vi "test_MonoAllTests.vi"(7 "Test should pass":bool=TRUE, 8 "error in":errorcluster, 9 "tear down connection":bool=TRUE, 10 "set-up a connection":bool=TRUE, 11 "device selection":enum16{"monochromator", "CCD", "SCD"}(ring)) -> (0 "error out":errorcluster)   [LabVIEW 2023]
uses:
  Classes/CCD/CCD.lvclass
  C:/Projects/Horiba/horiba-labview-sdk/Source/Classes/GenericDevice/GenericDevice.lvclass
  <vilib>/addons/_JKI Toolkits/Caraya/classes/Test/Test.lvclass
  <vilib>/Hampel Software Engineering/HSE Logger/hse-logger.lvlib
panel:
  in  "init mono?":bool
  out "log-file path":path
  # "Connector Pane"
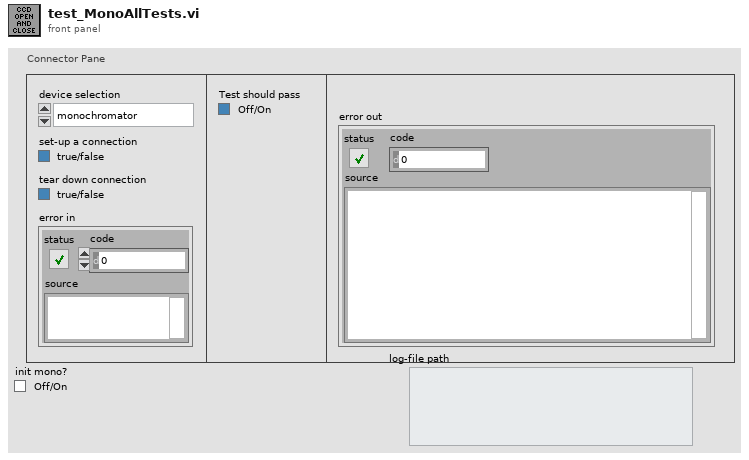
[diagram p1: front panel]
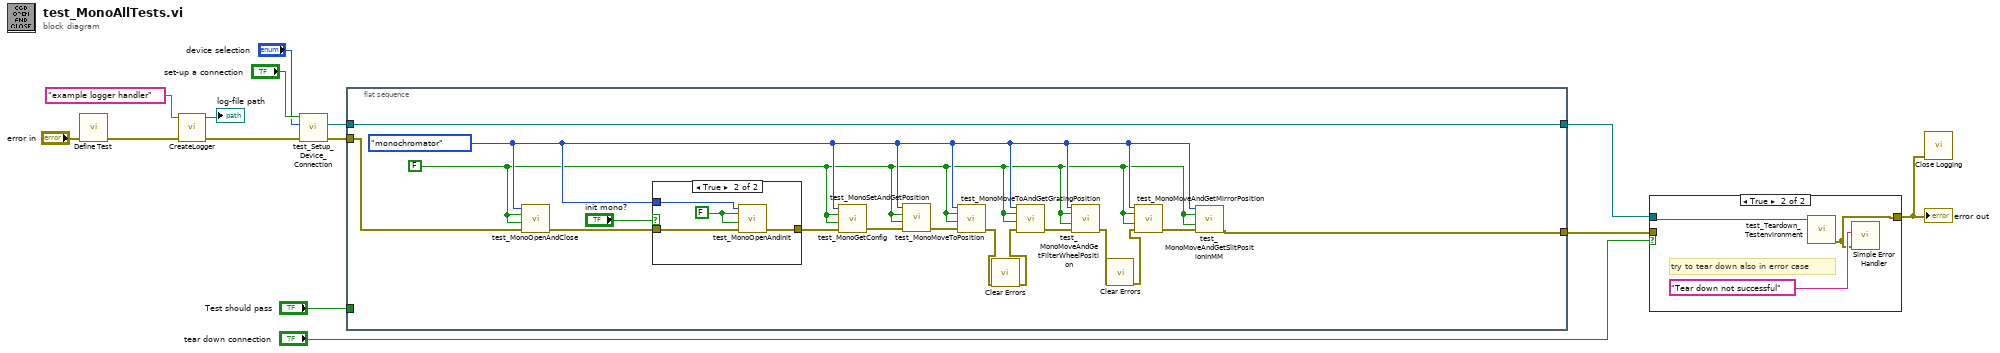
[diagram p0: block diagram]
diagram:
  n1 = call <vilib>:"Define Test.vi"("error in (no error)"="error in") -> ("error out"=w4:errorcluster)  [unwired: 9 in, 1 out]
  n2 = call "CreateLogger.vi"("error in (no error)"=w4, "Handler Name"="example logger handler") -> ("error out"=w3:errorcluster, "log-file path"=→"log-file path":path)  [unwired: 8 in]
  n3 = call "test_Setup_Device_Connection.vi"("error in (no error)"=w3, "device selection"="device selection", "set-up a connection"="set-up a connection") -> ("error out"=w7:errorcluster, "CCD.lvclass"=w8:refnum<class "CCD.lvclass">)  [unwired: 5 in, 2 out]
  n4 = flat-sequence {
    tunnel: w7 -> [w29]
    tunnel: w8 -> [w30]
    tunnel: "Test should pass" -> [_]
    tunnel: [w30] -> w11
    tunnel: [w19] -> w1
    frame #0 {
      w22 = enum16{"monochromator", "CCD", "SCD"}."monochromator" ("device selection")
      w21 = FALSE
      n5 = call "test_MonoOpenAndClose.vi"("error in"=w29, "tear down connection"=w21, "set-up a connection"=w21, "device selection"=w22) -> ("error out"=w27:errorcluster)  [unwired: 6 in, 1 out]
      n6 = case shown="True" "init mono?" {
        tunnel: w27 -> [w31 w35]
        tunnel: w22 -> [_ w33]
        tunnel: [w31 w32] -> w26
        frame False {
        }
        frame True {
          w34 = FALSE
          n7 = call "test_MonoOpenAndInit.vi"("error in"=w35, "tear down connection"=w34, "set-up a connection"=w34, "device selection"=w33) -> ("error out"=w32:errorcluster)  [unwired: 6 in, 1 out]
        }
      }
      n8 = call "test_MonoGetConfig.vi"("error in"=w26, "tear down connection"=w21, "set-up a connection"=w21, "device selection"=w22) -> ("error out"=w25:errorcluster)  [unwired: 7 in]
      n9 = call "test_MonoSetAndGetPosition.vi"("error in"=w25, "tear down connection"=w21, "set-up a connection"=w21, "device selection"=w22) -> ("error out"=w24:errorcluster)  [unwired: 6 in, 1 out]
      n10 = call "test_MonoMoveToPosition.vi"("device selection"=w22, "set-up a connection"=w21, "tear down connection"=w21, "error in"=w24) -> ("error out"=w18:errorcluster)  [unwired: 10 in, 1 out]
      n11 = call <vilib>:"Clear Errors.vi"("error in (no error)"=w18) -> ("error out"=w17:errorcluster)  [unwired: 5 in, 1 out]
      n12 = call "test_MonoMoveToAndGetGratingPosition.vi"("device selection"=w22, "set-up a connection"=w21, "tear down connection"=w21, "error in"=w17) -> ("error out"=w23:errorcluster)  [unwired: 10 in, 1 out]
      n13 = call "test_MonoMoveAndGetFilterWheelPosition.vi"("device selection"=w22, "set-up a connection"=w21, "tear down connection"=w21, "error in"=w23) -> ("error out"=w16:errorcluster)  [unwired: 10 in, 1 out]
      n14 = call <vilib>:"Clear Errors.vi"("error in (no error)"=w16) -> ("error out"=w15:errorcluster)  [unwired: 5 in, 1 out]
      n15 = call "test_MonoMoveAndGetMirrorPosition.vi"("device selection"=w22, "set-up a connection"=w21, "tear down connection"=w21, "error in"=w15) -> ("error out"=w20:errorcluster)  [unwired: 10 in, 1 out]
      n16 = call "test_MonoMoveAndGetSlitPositionInMM.vi"("device selection"=w22, "set-up a connection"=w21, "tear down connection"=w21, "error in"=w20) -> ("error out"=w19:errorcluster)  [unwired: 10 in, 1 out]
    }
  }
  n17 = case shown="True" "tear down connection" {
    tunnel: w11 -> [_ w38]
    tunnel: [w36 w37] -> w2
    tunnel: w1 -> [w36 _]
    frame False {
    }
    frame True {
      # "try to tear down also in error case"
      n18 = call "test_Teardown_Testenvironment.vi"("GenericDevice.lvclass"=w38) -> ("error out"=w37:errorcluster)  [unwired: 9 in, 1 out]
      n19 = call <vilib>:"Simple Error Handler.vi"("error source (\" \")"="Tear down not successful" ("error source (\" \")"), "error in (no error)"=w37) -> ()  [unwired: 3 in, 5 out]
    }
  }
  "error out" <- w2
  n20 = call <vilib>:"Close Logging.vi"("error in"=w2) -> ()  [unwired: 10 in, 1 out]
